vi "niDTS GNSS Dut Rx Fetch Results.vi"(0 "Dut Handle in":T2, 11 "error in (no error)":errorcluster) -> (4 "Dut Handle out":T2, 8 "Results":T1, 15 "error out":errorcluster)   [LabVIEW 2015, in "niDTS GNSS.lvlib"]
uses:
  niDTS GNSS.lvlib
  Framework/Dut/Includes/niDTS Dut INC Handle.ctl
  Framework/Dut/Objects/BASE_class/niDTS Dut.lvclass
  Tests/RF Test/Includes/niDTS GNSS RF Test INC Results.ctl
  Includes/niDTS GNSS Dut INC Handle.ctl
  Objects/BASE_class/niDTS GNSS Dut.lvclass
  Framework/niDTS Framework.lvlib
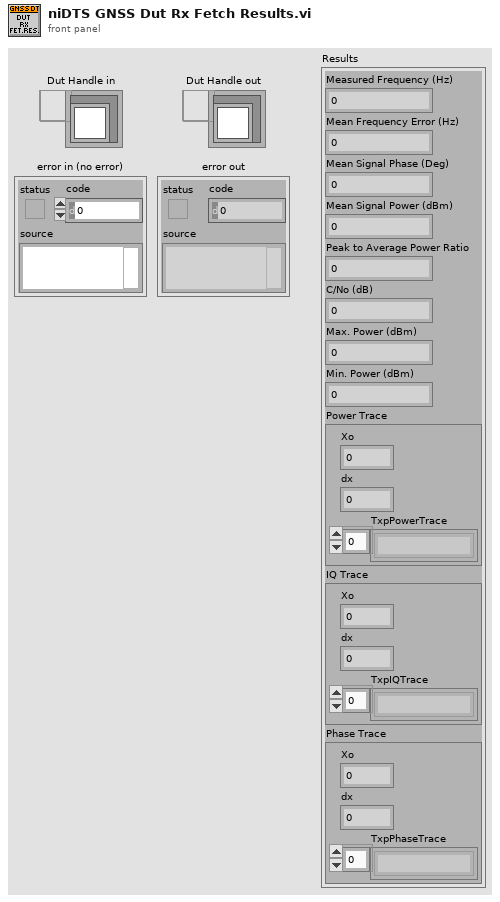
[diagram p1: front panel]
types:
  T1 = typedef "niDTS GNSS.lvlib/niDTS GNSS RF Test INC Results.ctl" = cluster{"Measured Frequency (Hz)":dbl, "Mean Frequency Error (Hz)":dbl, "Mean Signal Phase (Deg)":dbl, "Mean Signal Power (dBm)":dbl, "Peak to Average Power Ratio":dbl, "C/No (dB)":dbl, "Max. Power (dBm)":dbl, "Min. Power (dBm)":dbl, "Power Trace":cluster{"Xo":dbl, "dx":dbl, "TxpPowerTrace":string[]}, "IQ Trace":cluster{"Xo":dbl, "dx":dbl, "TxpIQTrace":string[]}, "Phase Trace":cluster{"Xo":dbl, "dx":dbl, "TxpPhaseTrace":string[]}}
  T2 = typedef "niDTS Framework.lvlib/niDTS Dut INC Handle.ctl" = refnum<data-value>
  T3 = typedef "niDTS GNSS.lvlib/niDTS GNSS Dut INC Handle.ctl" = refnum<data-value>
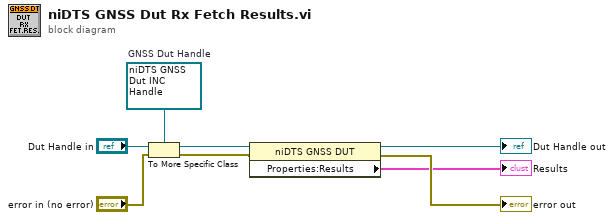
[diagram p0: block diagram]
diagram:
  w6 = T3 refnum  # GNSS Dut Handle
  n1 = To More Specific Class(target class=w6, reference="Dut Handle in", error in="error in (no error)") -> (specific class reference=w5:T3, error out=w4:errorcluster)
  n2 = property class="niDTS GNSS DUT"(reference=w5, error in=w4) -> (reference out=→"Dut Handle out":T3, error out=→"error out":errorcluster, "Properties:Results"=→"Results":T1)
